vi "EMV Detect Flow Stop.vi"(0 "History Input":dbl[](array[numeric]), 1 "Position?":bool, 2 "Flow State (0x4009)":u8, 5 "Input":T2, 7 "T6":dbl, 11 "error in (no error)":errorcluster, 12 "User Setpoint (0x4024)":u16, 13 "Est. Temp Rise":dbl=1.5 format="%#_13g") -> (4 "Current T7 Temperatures Output":dbl[](array[numeric]), 6 "Output":T2, 15 "error out":errorcluster)   [LabVIEW 2016]
uses:
  type defs/EMV Flow Stop Detection.ctl
panel:
  in  "Enum":T1(ring)=enum."Simple"
  out "Upper Limit":dbl
  in  "Sigma":dbl=4.0 format="%#_13g"
  in  "T7_DELTA_FLOW_THRESHOLD":dbl
  out "Slope Chart":dbl(graph)
  in  "Abnormal Input Temperature":dbl=90.0
  in  "T7_DELTA_INDICATING_FLOW":dbl
  in  "Cold Water Supply Temperature":dbl
  in  "Detection Slope":dbl=0.2 format="%#_13g"
  in  "T7 STOP-T6 FLOW -THRESHOLD":dbl
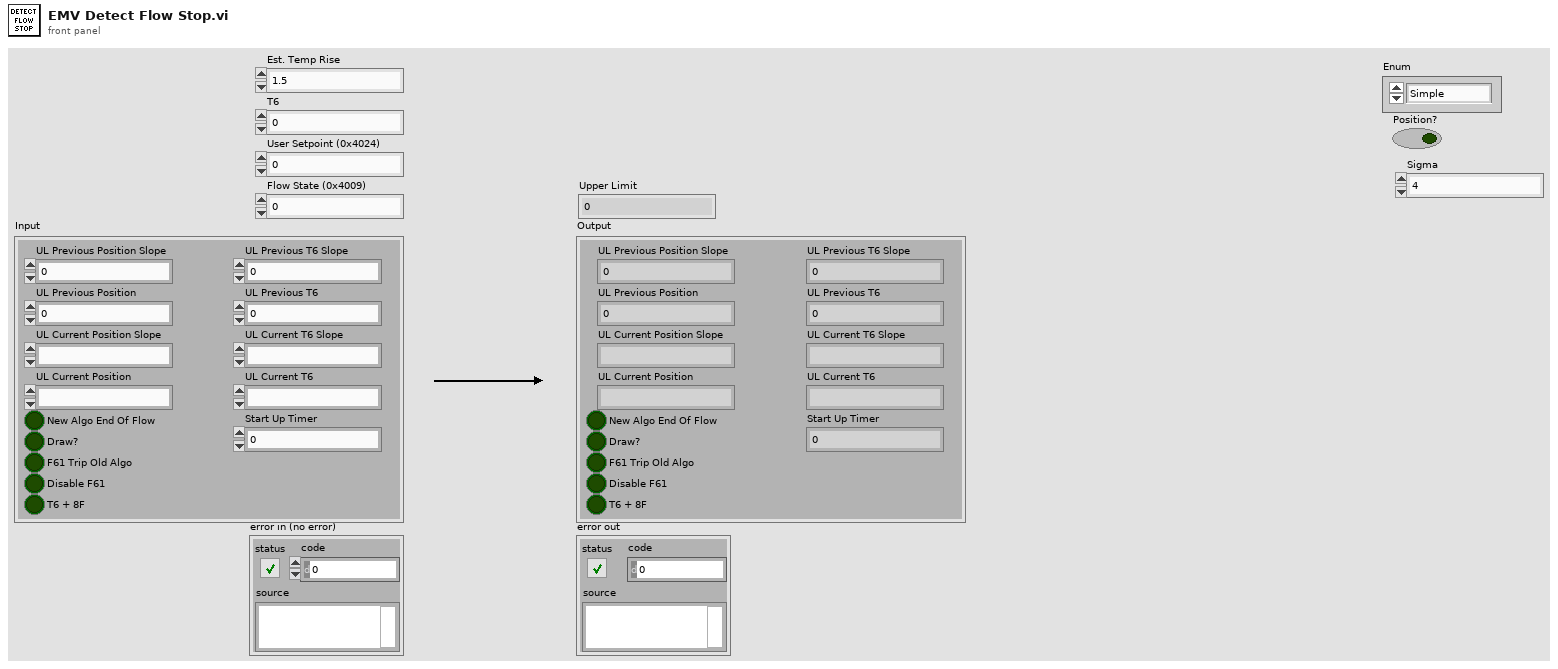
[diagram p1: front panel]
types:
  T1 = enum16{"End Slope", "Complex Slope Algo", "Simple"}
  T2 = typedef "EMV Flow Stop Detection.ctl" = cluster{"UL Previous Position Slope":dbl, "UL Previous T6 Slope":dbl, "UL Previous Position":dbl, "UL Previous T6":dbl, "UL Current Position":dbl, "UL Current Position Slope":dbl, "UL Current T6":dbl, "UL Current T6 Slope":dbl, "New Algo End Of Flow":bool, "Start Up Timer":dbl, "Draw?":bool, "Disable F61":bool, "F61 Trip Old Algo":bool, "T6 + 8F":bool}
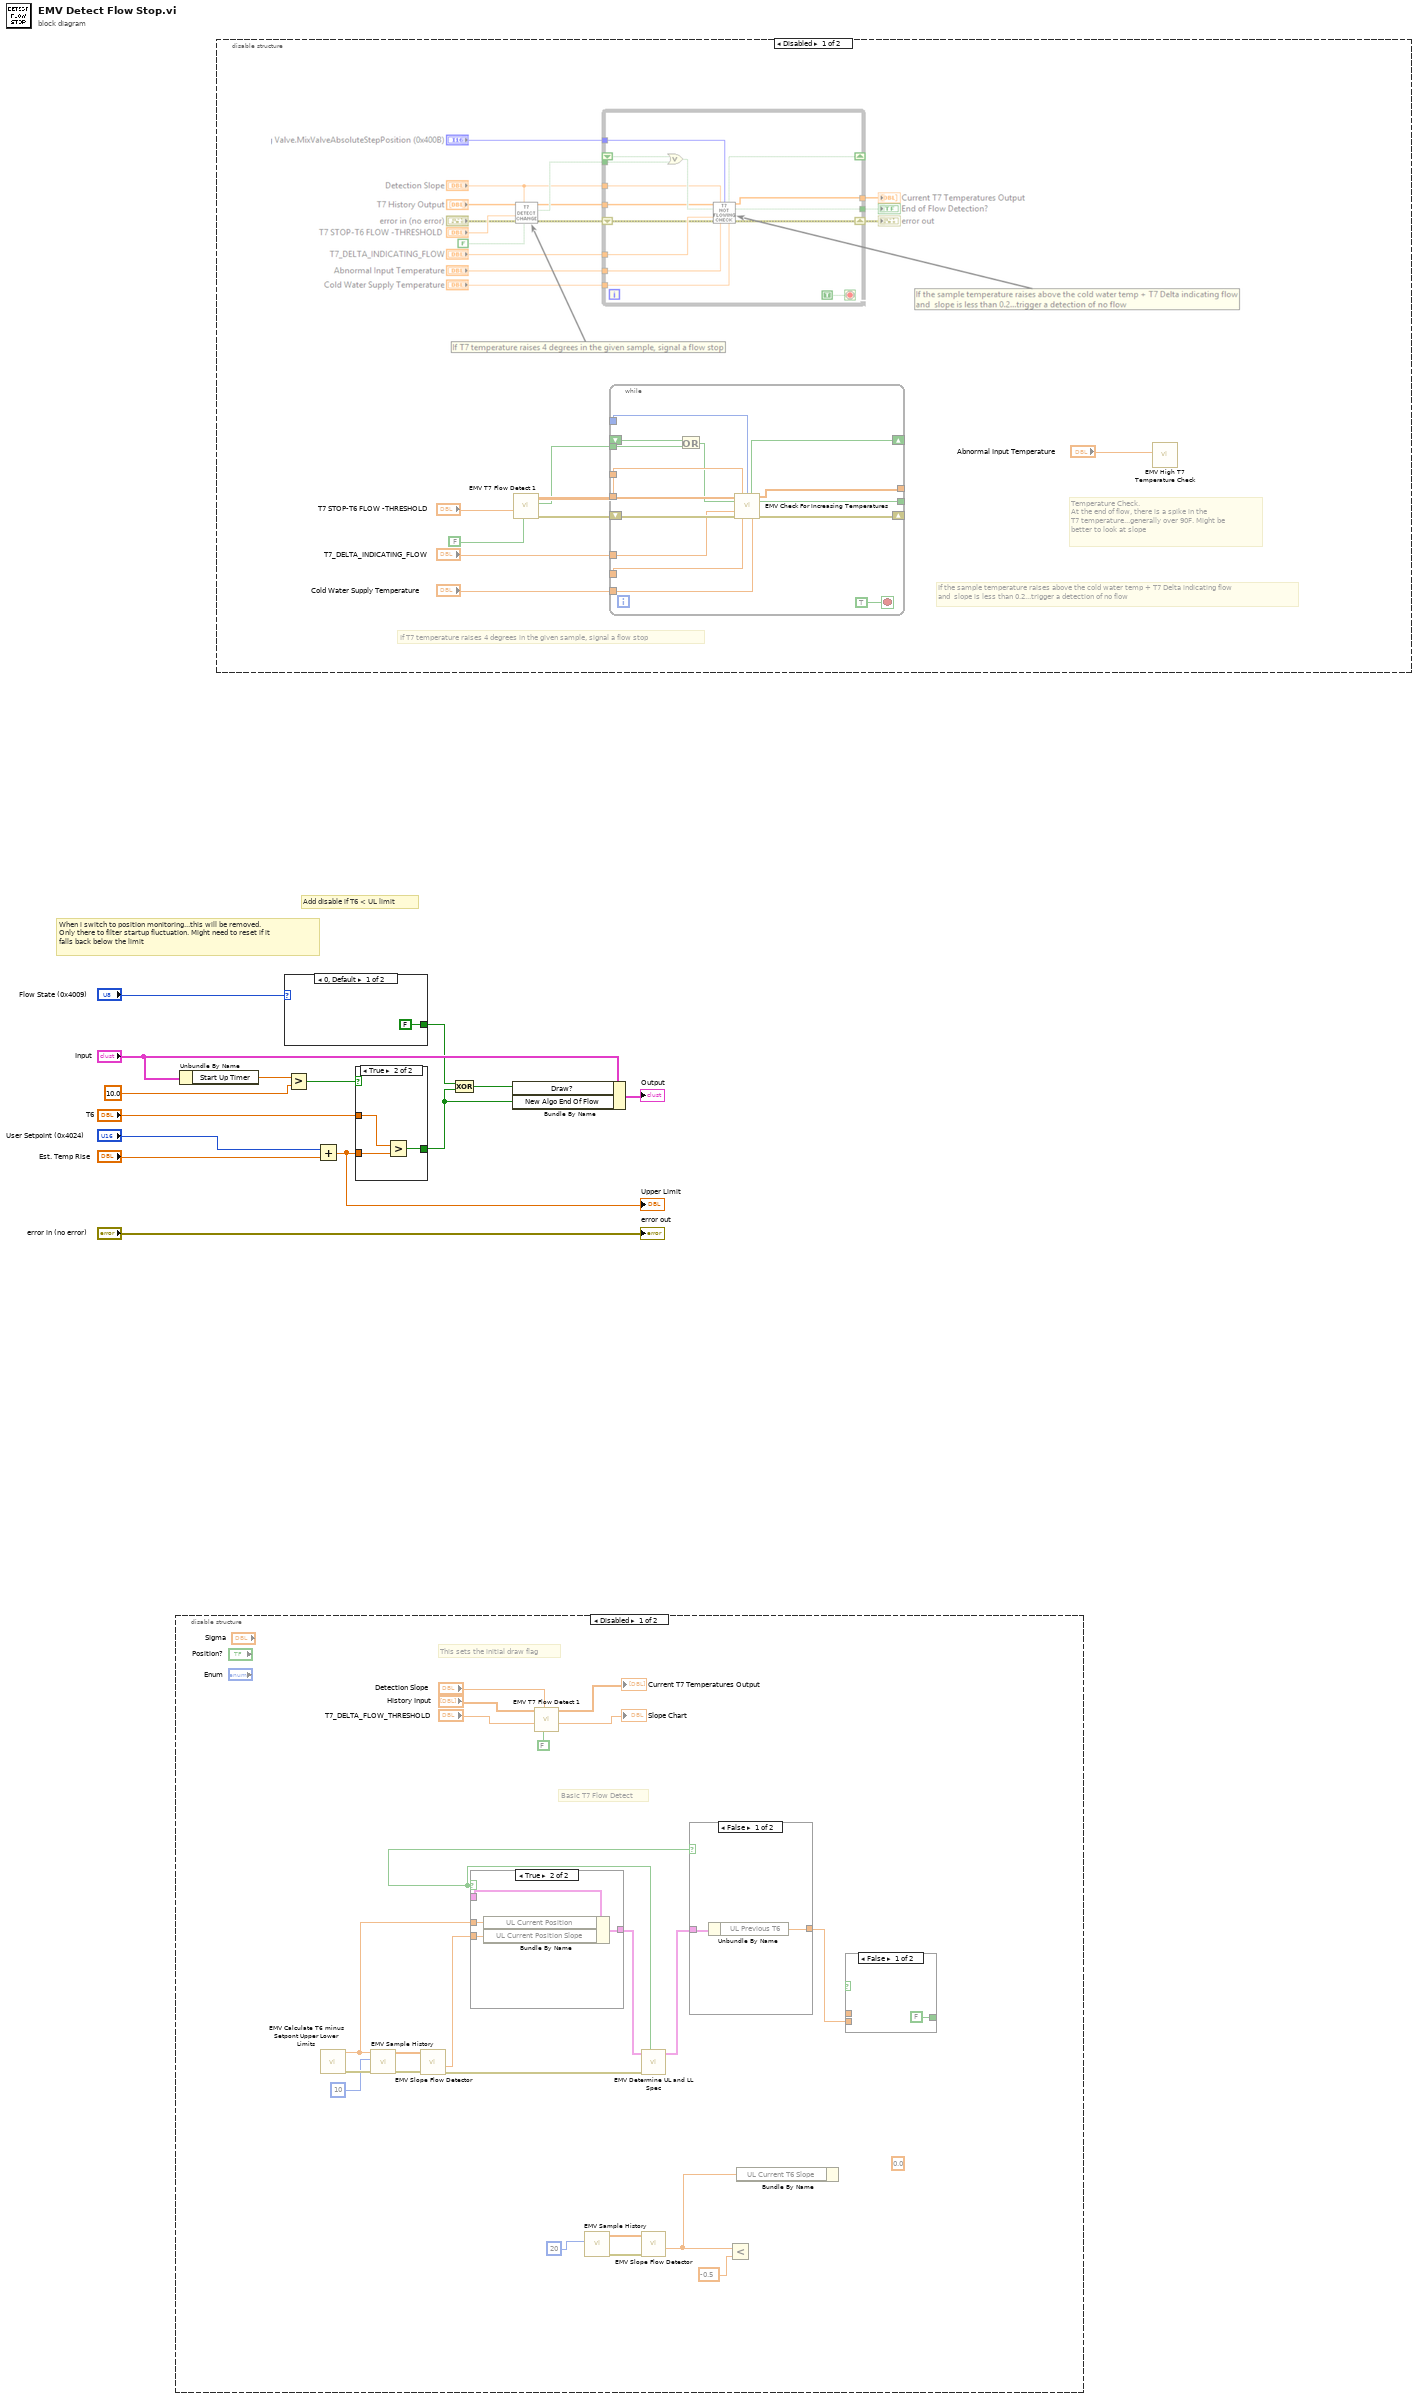
[diagram p0: block diagram]
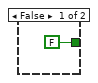
[diagram p2: hidden frame]
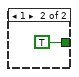
[diagram p3: hidden frame]
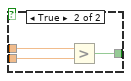
[diagram p4: hidden frame]
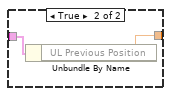
[diagram p5: hidden frame]
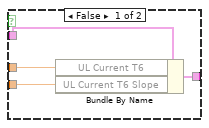
[diagram p6: hidden frame]
diagram:
  # "Add disable if T6 < UL limit"
  # "When i switch to position monitoring...this will be removed.\nOnly there to filter startup fluctuation. Might need to reset if it\nfalls back below the limit"
  n1 = disable-structure shown="Disabled" {
    frame Disabled {
      w23 = 0.0 ("UL Previous Position")
      # "Basic T7 Flow Detect"
      # "This sets the initial draw flag"
      n2 = call "EMV Calculate T6 minus Setpont Upper Lower Limits.vi"() -> ("error out"=w32:errorcluster, "Upper Limit"=w35:dbl, "error in (no error)"=w38:errorcluster, "Sigma"=w27:dbl)  [unwired: 7 in, 1 out]
      n3 = call "EMV Sample History.vi"("error in (no error)"=w32, "length"=10, "T6 Temp"=w35) -> ("error out"=w30:errorcluster, "T6 History"=w29:dbl[])  [unwired: 7 in]
      n4 = call "EMV Slope Flow Detector.vi"("error in (no error)"=w30, "Current T6 Temperatures in"=w29) -> ("error out"=w31:errorcluster, "slope"=w36:dbl)  [unwired: 7 in, 1 out]
      n5 = case shown="True" w37 {
        tunnel: [w61 w64] -> w33
        tunnel: [w60 w65] -> w34
        tunnel: w35 -> [w59 w62]
        tunnel: w36 -> [w58 w63]
        frame False {
          n6 = Bundle By Name(cluster=w61, "UL Current T6"=w59, "UL Current T6 Slope"=w58) -> (w60:cluster{})
        }
        frame True {
          n7 = Bundle By Name(cluster=w64, "UL Current Position"=w62, "UL Current Position Slope"=w63) -> (w65:cluster{})
        }
      }
      n8 = call "EMV T7 Flow Detect 1.vi"("Detect Flow Start?"=FALSE, "Detection Slope"="Detection Slope", "T7_DELTA_FLOW_THRESHOLD"="T7_DELTA_FLOW_THRESHOLD", "Current T7 Temperatures"="History Input") -> ("slope"=→"Slope Chart":dbl, "Current T7 Temperatures Output"=→"Current T7 Temperatures Output":dbl[])  [unwired: 4 in, 2 out]
      n9 = call "EMV Sample History.vi"("length"=20) -> ("error out"=w21:errorcluster, "T6 History"=w22:dbl[], "error in (no error)"=w25:errorcluster, "T6 Temp"=w24:dbl)  [unwired: 7 in]
      n10 = call "EMV Determine UL and LL Spec.vi"("Position?"=w37, "error in (no error)"=w31, "Input"=w34) -> ("error out"=w39:errorcluster, "Output"=w40:T2)  [unwired: 7 in]
      n11 = call "EMV Slope Flow Detector.vi"("error in (no error)"=w21, "Current T6 Temperatures in"=w22) -> ("error out"=w20:errorcluster, "slope"=w15:dbl)  [unwired: 7 in, 1 out]
      n12 = case shown="False" w37 {
        tunnel: w40 -> [w55 w57]
        tunnel: [w54 w56] -> w41
        frame False {
          n13 = Unbundle By Name(w55) -> ("UL Previous T6"=w54:dbl)
        }
        frame True {
          n14 = Unbundle By Name(w57) -> ("UL Previous Position"=w56:dbl)
        }
      }
      n15 = Less?(x=w15, y=-0.5) -> (x < y?=w18:bool)
      n16 = Bundle By Name("UL Current T6 Slope"=w15) -> (w16:cluster{}, w17:cluster{})
      n17 = case shown="False" w43 {
        tunnel: [_ w53] -> w42
        tunnel: w41 -> [_ w52]
        tunnel: [FALSE w51] -> _
        frame False {
        }
        frame True {
          n18 = Greater?(x=w53, y=w52) -> (0:w51:bool)
        }
      }
    }
    frame Enabled {
    }
  }
  n19 = Unbundle By Name("Input") -> ("Start Up Timer"=w10:dbl)
  n20 = disable-structure shown="Disabled" {
    frame Disabled {
      # "Temperature Check.\nAt the end of flow, there is a spike in the \nT7 temperature...generally over 90F. Might be\nbetter to look at slope"
      # "If the sample temperature raises above the cold water temp + T7 Delta indicating flow\nand  slope is less than 0.2...trigger a detection of no flow"
      # "If T7 temperature raises 4 degrees in the given sample, signal a flow stop"
      n21 = call "EMV T7 Flow Detect 1.vi"("Detect Flow Start?"=FALSE, "T7_DELTA_FLOW_THRESHOLD"="T7 STOP-T6 FLOW -THRESHOLD") -> ("error out"=w71:errorcluster, "Detection?"=w67:bool, "Current T7 Temperatures Output"=w68:dbl[], "Detection Slope"=w69:dbl)  [unwired: 5 in, 1 out]
      n22 = while {
        tunnel: "Cold Water Supply Temperature" -> [w89]
        tunnel: "T7_DELTA_INDICATING_FLOW" -> [w79]
        tunnel: [w86] -> _
        tunnel: w69 -> [w85]
        tunnel: w68 -> [w84]
        shift-right: [w88] -> _
        shift-left: w71 -> [w87]
        shift-right: [w82] -> _
        shift-left: _ -> [w81]
        tunnel: w67 -> [w80]
        tunnel: _ -> [w77]
        tunnel: _ -> [w76]
        tunnel: [w75] -> _
        stop <- TRUE stop-if-true
        n23 = Or(x=w81, y=w80) -> (x .or. y?=w78:bool)
        n24 = call "EMV Check For Increasing Temperatures.vi"("Current T7 Temperatures"=w84, "Detection Slope"=w85, "Mixing Valve.MixValveAbsoluteStepPosition (0x400B)"=w76, "T7 Detection?"=w78, "T7_DELTA_INDICATING_FLOW"=w79, "error in (no error)"=w87, "Abnormal Input Temperature"=w77, "Cold Water Supply Temperature"=w89) -> ("Trigger Lock"=w82:bool, "Current T7 Temperatures Output"=w86:dbl[], "End of Flow Detection?"=w75:bool, "error out"=w88:errorcluster)  [unwired: 4 in]
      }
      n25 = call "EMV High T7 Temperature Check.vi"("Abnormal Input Temperature"="Abnormal Input Temperature") -> ()  [unwired: 8 in, 3 out]
    }
    frame Enabled {
    }
  }
  n26 = case shown="0, Default" "Flow State (0x4009)" {
    tunnel: [FALSE TRUE] -> w5
    frame 0, Default {
    }
    frame 1 {
    }
  }
  n27 = Greater?(x=w10, y=10.0 ("Counter")) -> (0:w3:bool)
  n28 = Add(x="User Setpoint (0x4024)", y="Est. Temp Rise") -> (x+y=w13:dbl)
  "Upper Limit" <- w13
  n29 = case shown="True" w3 {
    tunnel: "T6" -> [_ w95]
    tunnel: w13 -> [_ w94]
    tunnel: [FALSE w93] -> w2
    frame False {
    }
    frame True {
      n30 = Greater?(x=w95, y=w94) -> (0:w93:bool)
    }
  }
  n31 = Exclusive Or(1:w2, 2:w5) -> (0:w7:bool)
  n32 = Bundle By Name(cluster="Input", "Draw?"=w7, "New Algo End Of Flow"=w2) -> (→"Output":T2)
  "error out" <- "error in (no error)"
